vi "Motor Sets (SubVI).vi"() -> ()   [LabVIEW 2020]
uses:
  <vilib>/Rock Robotics/WPI/ThirdParty/Phoenix-LabVIEW/Motor Controller/Controls/CTRE_Phoenix_MotorControl_ControlMode.ctl
  <vilib>/Rock Robotics/WPI/ThirdParty/REV Robotics/REVLib/Typedef/Spark MAX Control Type.ctl
  <vilib>/Rock Robotics/WPI/ThirdParty/REV Robotics/REVLib/Typedef/Spark MAX Idle Mode.ctl
  Team Code/Robot Global Data.vi
  <vilib>/Rock Robotics/WPI/ThirdParty/Phoenix-LabVIEW/Motor Controller/Get/CTRE_Phoenix_MotorController_IntegratedSensorData_TalonFX.vi
  <vilib>/Rock Robotics/WPI/ThirdParty/Phoenix-LabVIEW/Motor Controller/Get/CTRE_Phoenix_MotorController_GetSelectedSensorData.vi
panel:
  in  "servoOverride":bool
  in  "servoPosition":dbl
  out "climerArmOutput":dbl
  in  "climberWinchOverride":bool
  in  "winchMode":T1=2 items=["PercentOutput"=0, "Position"=1, "Velocity"=2, "Current"=3, "Follower"=5, "MotionProfile"=6, "MotionMagic"=7, "MotionProfileArc"=10, "Disabled"=15]
  in  "winchOutput":dbl
  in  "kFWinch":dbl
  in  "kPWinch":dbl=0.06
  in  "kDWinch":dbl
  in  "climberWinchPIDOverride":bool
  out "climberWinch":dbl(graph)
  in  "climberArmOverride":bool
  out "climberArmPosition":dbl(graph)
  in  "climberArmControlMode":T2=enum."Position"
  in  "climberArmPosition":dbl
  in  "climberArmPIDConstants":T3={"P Gain"=0.01, "I Gain"=0.0, "D Gain"=0.0, "F Gain"=0.0, "I Zone"=0.0, "Min Output"=-0.5, "Max Output"=0.5}
  in  "climberArmPIDOveride":bool
  in  "intakeLift":bool
  out "intakeLiftPosition":dbl(graph)
  in  "intakeLiftControlMode":T2=enum."Position"
  in  "intakeLiftPosition":dbl
  in  "intakeLiftPIDConstants":T3={"P Gain"=0.0025, "I Gain"=0.0, "D Gain"=1.0, "F Gain"=0.0, "I Zone"=0.0, "Min Output"=-0.7, "Max Output"=0.7}
  in  "intakeLiftPIDOveride":bool
  in  "leftShooterOutput":dbl
  in  "intakeOverride":bool
  in  "intakeMode":T1 items=["PercentOutput"=0, "Position"=1, "Velocity"=2, "Current"=3, "Follower"=5, "MotionProfile"=6, "MotionMagic"=7, "MotionProfileArc"=10, "Disabled"=15]
  in  "intakeOutput":dbl
  in  "kFIntake":dbl=0.0491
  in  "kPIntake":dbl=0.06
  in  "kDIntake":dbl=5.0
  in  "intakePIDOverride":bool
  out "intake":i32(graph)
  out "turretAngle Position":dbl
  out "turretAngle":dbl(graph)
  in  "Turret PID Constants":T3={"P Gain"=0.0, "I Gain"=0.0, "D Gain"=0.0, "F Gain"=0.0, "I Zone"=0.0, "Min Output"=-1.0, "Max Output"=1.0}
  in  "hoodPIDOverride":bool
  in  "turretControlMotor":T2=enum."Position"
  in  "hoodPosition":dbl
  in  "PID Constants":T3={"P Gain"=0.009, "I Gain"=0.0, "D Gain"=0.0, "F Gain"=0.0, "I Zone"=0.0, "Min Output"=-0.6, "Max Output"=0.6}
  in  "Control Mode":T2=enum."Position"
  in  "kDShooter":dbl=2.0
  in  "kDKickup":dbl=5.0
  out "LoopTime (ms)":u32
  out "hoodAngle":dbl(graph)
  out "kickup":i32(graph)
  out "leftShooter":i32(graph)
  out "rightShooter":i32(graph)
  in  "turretAnglePIDOverride":bool
  in  "kickupPIDOverride":bool
  in  "kFKickup":dbl=0.0491
  in  "kPKickup":dbl=0.06
  in  "kPShooter":dbl=0.3
  in  "kFShooter":dbl=0.0506
  in  "shooterPIDOverride":bool
  in  "righrRearDriveOutput":dbl
  in  "leftRearDriveOutput":dbl
  in  "rightFrontDriveOutput":dbl
  out "rightRearDriveVelocity":i32(graph)
  out "leftRearDriveVelocity":i32(graph)
  out "rightFrontDriveVelocity":i32(graph)
  out "leftFrontDriveVelocity":i32(graph)
  in  "KdDrive":dbl
  in  "KpDrive":dbl
  in  "drivePIDOverride":bool
  in  "turretAngleOutput":dbl
  in  "turretAngleOverride":bool
  in  "hoodAngleOverride":bool
  in  "steeringMotorOverride":bool
  in  "rightRearSteeringOutput":dbl
  in  "leftRearSteeringOutput":dbl
  in  "rightFrontSteeringOutput":dbl
  in  "leftFrontSteeringOutput":dbl
  in  "indexerOutput":dbl
  in  "indexOverride":bool
  in  "driveMode":T1=2 items=["PercentOutput"=0, "Position"=1, "Velocity"=2, "Current"=3, "Follower"=5, "MotionProfile"=6, "MotionMagic"=7, "MotionProfileArc"=10, "Disabled"=15]
  in  "rightShooterOutput":dbl
  in  "shooterMode":T1=2 items=["PercentOutput"=0, "Position"=1, "Velocity"=2, "Current"=3, "Follower"=5, "MotionProfile"=6, "MotionMagic"=7, "MotionProfileArc"=10, "Disabled"=15]
  in  "shooterOverride":bool
  in  "kickupOutput":dbl
  in  "kickupMode":T1=2 items=["PercentOutput"=0, "Position"=1, "Velocity"=2, "Current"=3, "Follower"=5, "MotionProfile"=6, "MotionMagic"=7, "MotionProfileArc"=10, "Disabled"=15]
  in  "kickupOverride":bool
  in  "leftFrontDriveOutput":dbl
  in  "driveOverride":bool
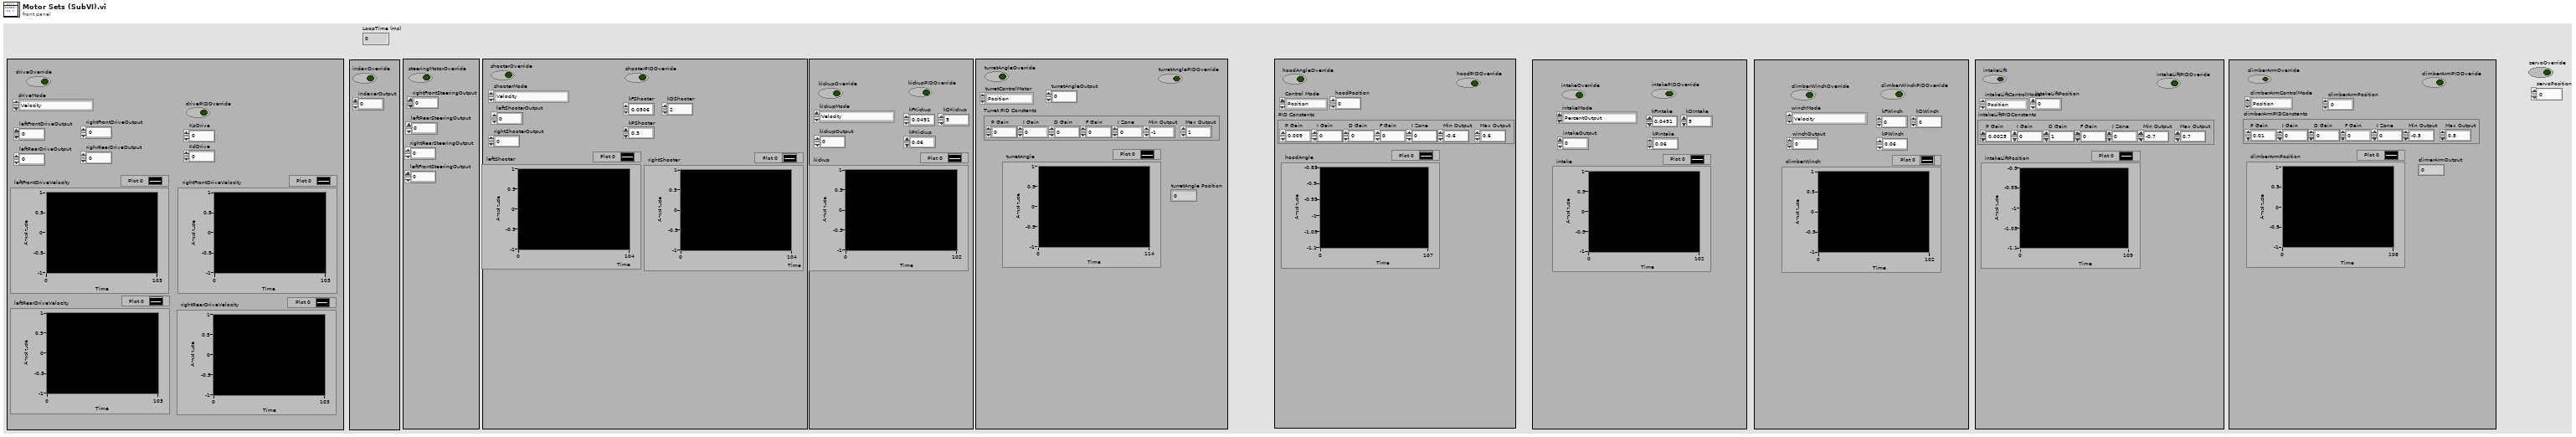
[diagram p1: front panel]
types:
  T1 = typedef "CTRE_Phoenix_MotorControl_ControlMode.ctl" = u16
  T2 = typedef "Spark MAX Control Type.ctl" = enum16{"Percent VBus", "Voltage", "Velocity", "Position", "Smart Motion", "Current", "Smart Velocity"}
  T3 = cluster{"P Gain":dbl, "I Gain":dbl, "D Gain":dbl, "F Gain":dbl, "I Zone":dbl, "Min Output":dbl, "Max Output":dbl}
  T4 = typedef "WPI_MotorControlDeviceRef.ctl" = cluster{"DeviceStatus":errorcluster, "Type":T5, "PWM":cluster{"PWM Channel":T6, "DeadBand":T7}, "CAN":cluster{"Device Number":u8, "SetOutput VI Ref":variant, "GetOutput VI Ref":variant, "Enable VI Ref":variant, "Disable VI Ref":variant, "Data":variant}, "Invert":bool, "DIO PWM":cluster{"PWM \"Enable\" Channel":T6, "DIOChannel":T8, "PWM Rate":dbl}}
  T5 = typedef "WPI_MotorControlType.ctl" = enum16{"PWM", "CAN", "DIO PWM"}
  T6 = typedef "FPGA_DIOPWMChannel.ctl" = enum8{"PWM 0", "PWM 1", "PWM 2", "PWM 3", "PWM 4", "PWM 5", "PWM 6", "PWM 7", "PWM 8", "PWM 9", "PWM MXP 0", "PWM MXP 1", "PWM MXP 2", "PWM MXP 3", "PWM MXP 4", "PWM MXP 5", "PWM MXP 6", "PWM MXP 7", "PWM MXP 8", "PWM MXP 9", "Invalid"}
  T7 = typedef "WPI_PWMDeadband.ctl" = cluster{"Name":string, "maxPositivePwm":i32, "minPositivePwm":i32, "centerPwm":i32, "maxNegativePwm":i32, "minNegativePwm":i32, "angularRange":u16}
  T8 = typedef "FPGA_DIOChannel.ctl" = enum8{"DIO 0", "DIO 1", "DIO 2", "DIO 3", "DIO 4", "DIO 5", "DIO 6", "DIO 7", "DIO 8", "DIO 9", "DIO MXP 0", "DIO MXP 1", "DIO MXP 2", "DIO MXP 3", "DIO MXP 4", "DIO MXP 5", "DIO MXP 6", "DIO MXP 7", "DIO MXP 8", "DIO MXP 9", "DIO MXP 10", "DIO MXP 11", "DIO MXP 12", "DIO MXP 13", "DIO MXP 14", "DIO MXP 15", "SPI Port CS1", "SPI Port CS2", "SPI Port CS3", "SPI Port MISO", "SPI Port MOSI", "Invalid"}
  T9 = typedef "WPI_ServoDeviceRef.ctl" = cluster{"DeviceStatus":errorcluster, "PWM Channel":T6, "DeadBand":T7}
  T10 = typedef "Spark MAX Idle Mode.ctl" = enum16{"Coast", "Brake"}
  T11 = cluster{"leftFrontDesiredVelocity":dbl, "leftRearDesiredVelocity":dbl, "rightFrontDesiredVelocity":dbl, "rightRearDesiredVelocity":dbl}
  T12 = cluster{"leftFrontSteeringPower":dbl, "leftRearSteeringPower":dbl, "rightFrontSteeringPower":dbl, "rightRearSteeringPower":dbl}
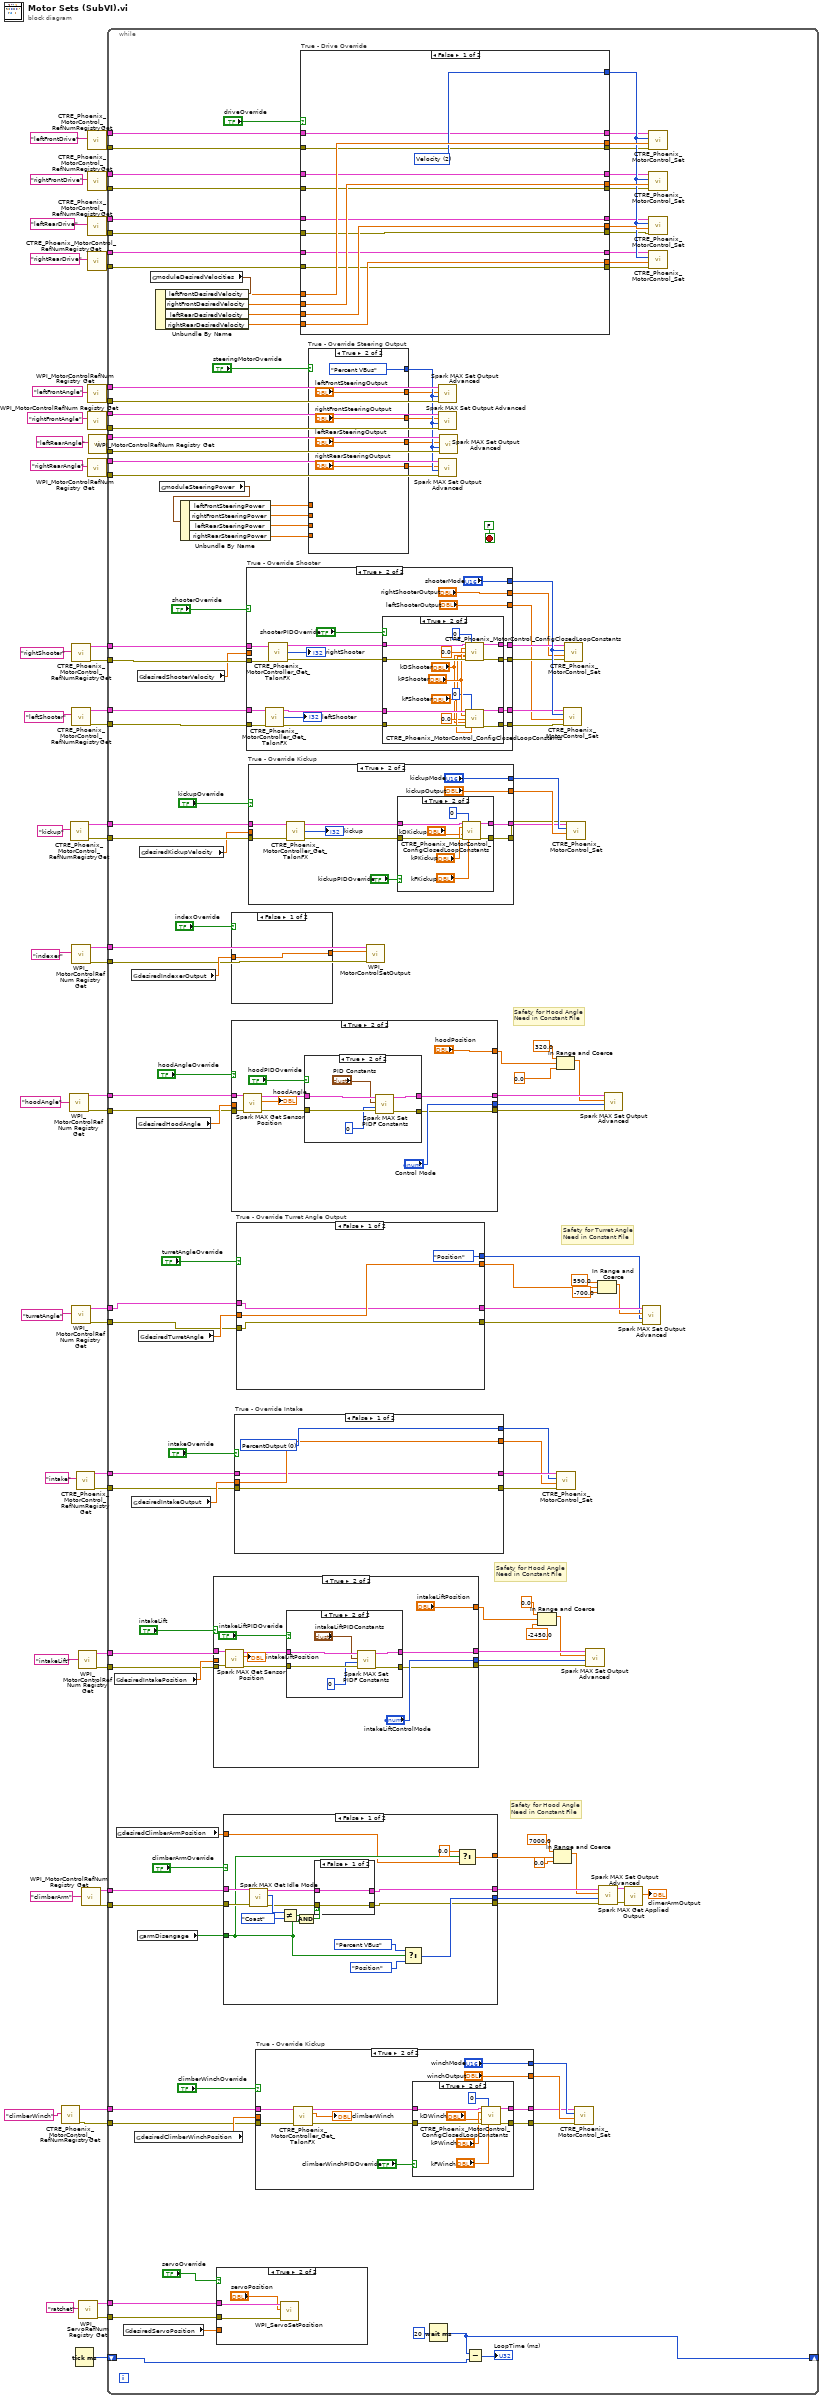
[diagram p0: block diagram]
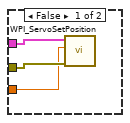
[diagram p2: hidden frame]
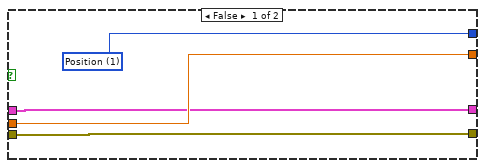
[diagram p3: hidden frame]
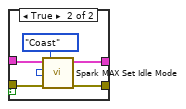
[diagram p5: hidden frame]
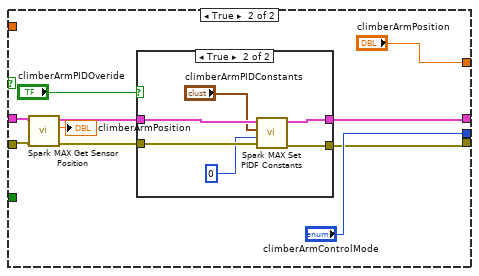
[diagram p6: hidden frame]
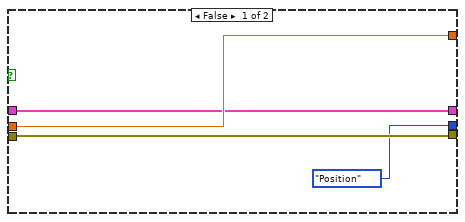
[diagram p8: hidden frame]
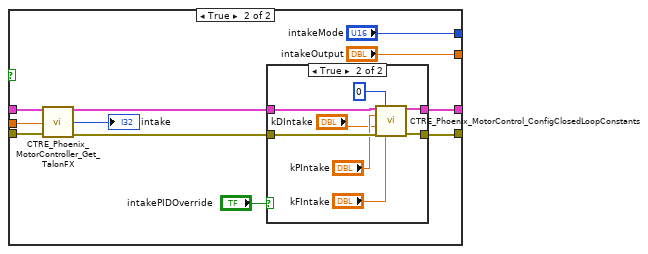
[diagram p10: hidden frame]
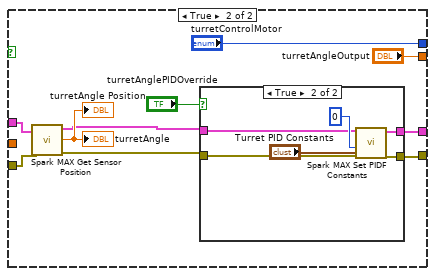
[diagram p12: hidden frame]
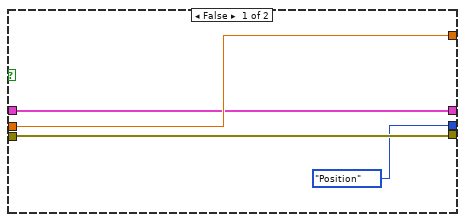
[diagram p14: hidden frame]
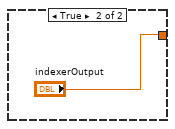
[diagram p16: hidden frame]
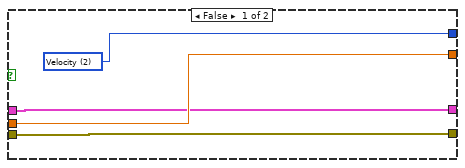
[diagram p17: hidden frame]
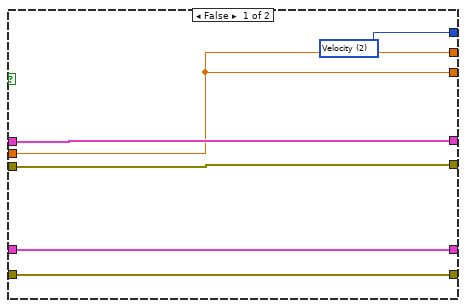
[diagram p19: hidden frame]
diagram:
  n1 = call <vilib>:"CTRE_Phoenix_MotorControl_RefNumRegistryGet.vi"("refnum name"="climberWinch") -> ("error out"=w4:errorcluster, "PhoenixMotorControlDevRef"=w5:T4)  [unwired: 9 in]
  n2 = call <vilib>:"WPI_MotorControlRefNum Registry Get.vi"("refnum name"="hoodAngle") -> ("error out"=w22:errorcluster, "MotorControlDevRef"=w23:T4)  [unwired: 9 in]
  n3 = call <vilib>:"CTRE_Phoenix_MotorControl_RefNumRegistryGet.vi"("refnum name"="kickup") -> ("error out"=w28:errorcluster, "PhoenixMotorControlDevRef"=w27:T4)  [unwired: 9 in]
  n4 = call <vilib>:"CTRE_Phoenix_MotorControl_RefNumRegistryGet.vi"("refnum name"="rightShooter") -> ("error out"=w30:errorcluster, "PhoenixMotorControlDevRef"=w29:T4)  [unwired: 9 in]
  n5 = call <vilib>:"CTRE_Phoenix_MotorControl_RefNumRegistryGet.vi"("refnum name"="leftShooter") -> ("error out"=w31:errorcluster, "PhoenixMotorControlDevRef"=w32:T4)  [unwired: 9 in]
  n6 = call <vilib>:"WPI_MotorControlRefNum Registry Get.vi"("refnum name"="indexer") -> ("error out"=w16:errorcluster, "MotorControlDevRef"=w17:T4)  [unwired: 9 in]
  n7 = call <vilib>:"WPI_MotorControlRefNum Registry Get.vi"("refnum name"="turretAngle") -> ("error out"=w19:errorcluster, "MotorControlDevRef"=w20:T4)  [unwired: 9 in]
  n8 = Tick Count (ms)() -> (millisecond timer value=w25:u32)
  n9 = call <vilib>:"CTRE_Phoenix_MotorControl_RefNumRegistryGet.vi"("refnum name"="intake") -> ("error out"=w13:errorcluster, "PhoenixMotorControlDevRef"=w14:T4)  [unwired: 9 in]
  n10 = call <vilib>:"WPI_MotorControlRefNum Registry Get.vi"("refnum name"="intakeLift") -> ("error out"=w10:errorcluster, "MotorControlDevRef"=w11:T4)  [unwired: 9 in]
  n11 = call <vilib>:"WPI_ServoRefNum Registry Get.vi"("refnum name"="ratchet") -> ("error out"=w1:errorcluster, "ServoDeviceRef"=w2:T9)  [unwired: 9 in]
  n12 = call <vilib>:"WPI_MotorControlRefNum Registry Get.vi"("refnum name"="climberArm") -> ("error out"=w7:errorcluster, "MotorControlDevRef"=w8:T4)  [unwired: 9 in]
  n13 = call <vilib>:"CTRE_Phoenix_MotorControl_RefNumRegistryGet.vi"("refnum name"="leftFrontDrive") -> ("error out"=w41:errorcluster, "PhoenixMotorControlDevRef"=w40:T4)  [unwired: 9 in]
  n14 = call <vilib>:"CTRE_Phoenix_MotorControl_RefNumRegistryGet.vi"("refnum name"="rightFrontDrive") -> ("error out"=w43:errorcluster, "PhoenixMotorControlDevRef"=w42:T4)  [unwired: 9 in]
  n15 = call <vilib>:"CTRE_Phoenix_MotorControl_RefNumRegistryGet.vi"("refnum name"="leftRearDrive") -> ("error out"=w45:errorcluster, "PhoenixMotorControlDevRef"=w44:T4)  [unwired: 9 in]
  n16 = call <vilib>:"CTRE_Phoenix_MotorControl_RefNumRegistryGet.vi"("refnum name"="rightRearDrive") -> ("error out"=w47:errorcluster, "PhoenixMotorControlDevRef"=w46:T4)  [unwired: 9 in]
  n17 = call <vilib>:"WPI_MotorControlRefNum Registry Get.vi"("refnum name"="leftFrontAngle") -> ("error out"=w49:errorcluster, "MotorControlDevRef"=w48:T4)  [unwired: 9 in]
  n18 = call <vilib>:"WPI_MotorControlRefNum Registry Get.vi"("refnum name"="rightFrontAngle") -> ("error out"=w50:errorcluster, "MotorControlDevRef"=w51:T4)  [unwired: 9 in]
  n19 = call <vilib>:"WPI_MotorControlRefNum Registry Get.vi"("refnum name"="rightRearAngle") -> ("error out"=w56:errorcluster, "MotorControlDevRef"=w57:T4)  [unwired: 9 in]
  n20 = call <vilib>:"WPI_MotorControlRefNum Registry Get.vi"("refnum name"="leftRearAngle") -> ("error out"=w55:errorcluster, "MotorControlDevRef"=w54:T4)  [unwired: 9 in]
  n21 = while {
    tunnel: w40 -> [w171]
    tunnel: w41 -> [w169]
    tunnel: w42 -> [w167]
    tunnel: w43 -> [w165]
    tunnel: w44 -> [w163]
    tunnel: w45 -> [w161]
    tunnel: w46 -> [w159]
    tunnel: w47 -> [w157]
    tunnel: w48 -> [w202]
    tunnel: w49 -> [w201]
    tunnel: w51 -> [w199]
    tunnel: w50 -> [w200]
    tunnel: w54 -> [w198]
    tunnel: w55 -> [w197]
    tunnel: w57 -> [w195]
    tunnel: w56 -> [w196]
    tunnel: w32 -> [w154]
    tunnel: w31 -> [w153]
    tunnel: w30 -> [w155]
    tunnel: w29 -> [w156]
    tunnel: w27 -> [w152]
    tunnel: w28 -> [w151]
    tunnel: w17 -> [w119]
    tunnel: w16 -> [w120]
    tunnel: w20 -> [w59]
    tunnel: w19 -> [w60]
    shift-right: [w147] -> _
    shift-left: w25 -> [w148]
    tunnel: w23 -> [w122]
    tunnel: w22 -> [w121]
    tunnel: w14 -> [w102]
    tunnel: w13 -> [w101]
    tunnel: w11 -> [w89]
    tunnel: w10 -> [w88]
    tunnel: w8 -> [w76]
    tunnel: w7 -> [w75]
    tunnel: w5 -> [w68]
    tunnel: w4 -> [w67]
    tunnel: w2 -> [w65]
    tunnel: w1 -> [w64]
    stop <- FALSE stop-if-true
    # "Safety for Hood Angle\nNeed in Constant File"
    # "Safety for Hood Angle\nNeed in Constant File"
    # "Safety for Turret Angle\nNeed in Constant File"
    # "Safety for Hood Angle\nNeed in Constant File"
    n22 = global read "Robot Global Data.vi" "desiredIntakePosition"() -> (w98:dbl)
    n23 = global read "Robot Global Data.vi" "desiredClimberArmPosition"() -> (w87:dbl)
    n24 = global read "Robot Global Data.vi" "desiredServoPosition"() -> (w62:dbl)
    n25 = global read "Robot Global Data.vi" "desiredIndexerOutput"() -> (w138:dbl)
    n26 = global read "Robot Global Data.vi" "desiredIntakeOutput"() -> (w104:dbl)
    n27 = global read "Robot Global Data.vi" "desiredClimberWinchPosition"() -> (w73:dbl)
    n28 = global read "Robot Global Data.vi" "desiredHoodAngle"() -> (w137:dbl)
    n29 = global read "Robot Global Data.vi" "desiredShooterVelocity"() -> (w145:dbl)
    n30 = global read "Robot Global Data.vi" "armDisengage"() -> (w61:bool)
    n31 = global read "Robot Global Data.vi" "desiredTurretAngle"() -> (w134:dbl)
    n32 = global read "Robot Global Data.vi" "desiredKickupVelocity"() -> (w143:dbl)
    n33 = global read "Robot Global Data.vi" "moduleDesiredVelocities"() -> (w192:T11)
    n34 = Unbundle By Name(w192) -> ("leftFrontDesiredVelocity"=w191:dbl, "rightFrontDesiredVelocity"=w190:dbl, "leftRearDesiredVelocity"=w189:dbl, "rightRearDesiredVelocity"=w188:dbl)
    n35 = global read "Robot Global Data.vi" "moduleSteeringPower"() -> (w193:T12)
    n36 = Unbundle By Name(w193) -> ("leftFrontSteeringPower"=w181:dbl, "rightFrontSteeringPower"=w180:dbl, "leftRearSteeringPower"=w179:dbl, "rightRearSteeringPower"=w178:dbl)
    n37 = case shown="True" "intakeLift" {
      tunnel: w98 -> [w279 _]
      tunnel: [w279 "intakeLiftPosition"] -> w96
      tunnel: w89 -> [w278 w280]
      tunnel: w88 -> [w277 w281]
      tunnel: [w277 w286] -> w92
      tunnel: [w278 w287] -> w93
      tunnel: [Spark_MAX_Control_Type."Position" ("Control Mode") "intakeLiftControlMode"] -> w90
      frame False {
      }
      frame True {
        n38 = call <vilib>:"Spark MAX Get Sensor Position.vi"("error in (no error)"=w281, "MotorControlDevRef in"=w280) -> ("error out"=w284:errorcluster, "Sensor Position"=→"intakeLiftPosition":dbl, "MotorControlDevRef out"=w285:T4)  [unwired: 6 in, 1 out]
        n39 = case shown="True" "intakeLiftPIDOveride" {
          tunnel: [w290 w297] -> w287
          tunnel: [w291 w296] -> w286
          tunnel: w285 -> [w290 w295]
          tunnel: w284 -> [w291 w294]
          frame False {
          }
          frame True {
            n40 = call <vilib>:"Spark MAX Set PIDF Constants.vi"("error in"=w294, "PIDF Slot"=0, "PID Constants"="intakeLiftPIDConstants", "MotorControlDeviceRef"=w295) -> ("error out"=w296:errorcluster, "MotorControlDeviceRef"=w297:T4)  [unwired: 6 in]
          }
        }
      }
    }
    n41 = case shown="True" "servoOverride" {
      tunnel: w65 -> [w206 w209]
      tunnel: w64 -> [w205 w208]
      tunnel: w62 -> [w204 _]
      frame False {
        n42 = call <vilib>:"WPI_ServoSetPosition.vi"("error in (no error)"=w205, "Position"=w204, "ServoDeviceRef"=w206) -> ()  [unwired: 7 in, 2 out]
      }
      frame True {
        n43 = call <vilib>:"WPI_ServoSetPosition.vi"("error in (no error)"=w208, "Position"="servoPosition", "ServoDeviceRef"=w209) -> ()  [unwired: 7 in, 2 out]
      }
    }
    n44 = case shown="False" "climberArmOverride" {
      tunnel: w87 -> [w235 _]
      tunnel: [w237 "climberArmPosition"] -> w85
      tunnel: w76 -> [w250 w258]
      tunnel: w75 -> [w249 w259]
      tunnel: [w238 w264] -> w79
      tunnel: [w239 w265] -> w80
      tunnel: [w242 "climberArmControlMode"] -> w77
      tunnel: w61 -> [w236 _]
      frame False {
        n45 = call <vilib>:"Spark MAX Get Idle Mode.vi"("error in (no error)"=w249, "MotorControlDeviceRef in"=w250) -> ("error out"=w243:errorcluster, "Idle Mode"=w248:T10, "MotorControlDeviceRef out"=w244:T4)  [unwired: 7 in]
        n46 = Not Equal?(x=w248, y=Spark_MAX_Idle_Mode."Coast") -> (x != y?=w246:bool)
        n47 = And(x=w246, y=w236) -> (x .and. y?=w245:bool)
        n48 = case shown="False" w245 {
          tunnel: w244 -> [w252 w256]
          tunnel: w243 -> [w251 w257]
          tunnel: [w252 w254] -> w239
          tunnel: [w251 w253] -> w238
          frame False {
          }
          frame True {
            n49 = call <vilib>:"Spark MAX Set Idle Mode.vi"("error in (no error)"=w257, "Idle Mode"=Spark_MAX_Idle_Mode."Coast", "MotorControlDeviceRef in"=w256) -> ("error out"=w253:errorcluster, "MotorControlDeviceRef out"=w254:T4)  [unwired: 7 in]
          }
        }
        n50 = Select(t=Spark_MAX_Control_Type."Percent VBus" ("Control Mode"), s=w236, f=Spark_MAX_Control_Type."Position" ("Control Mode")) -> (s? t:f=w242:T2)
        n51 = Select(t=0.0, s=w236, f=w235) -> (s? t:f=w237:dbl)
      }
      frame True {
        n52 = call <vilib>:"Spark MAX Get Sensor Position.vi"("error in (no error)"=w259, "MotorControlDevRef in"=w258) -> ("error out"=w262:errorcluster, "Sensor Position"=→"climberArmPosition":dbl, "MotorControlDevRef out"=w263:T4)  [unwired: 6 in, 1 out]
        n53 = case shown="True" "climberArmPIDOveride" {
          tunnel: [w268 w275] -> w265
          tunnel: [w269 w274] -> w264
          tunnel: w263 -> [w268 w273]
          tunnel: w262 -> [w269 w272]
          frame False {
          }
          frame True {
            n54 = call <vilib>:"Spark MAX Set PIDF Constants.vi"("error in"=w272, "PIDF Slot"=0, "PID Constants"="climberArmPIDConstants", "MotorControlDeviceRef"=w273) -> ("error out"=w274:errorcluster, "MotorControlDeviceRef"=w275:T4)  [unwired: 6 in]
          }
        }
      }
    }
    n55 = case shown="False" "indexOverride" {
      tunnel: w138 -> [w367 _]
      tunnel: [w367 "indexerOutput"] -> w118
      frame False {
      }
      frame True {
      }
    }
    n56 = case shown="True" "hoodAngleOverride" {
      tunnel: w137 -> [w348 _]
      tunnel: [w348 "hoodPosition"] -> w127
      tunnel: w122 -> [w347 w358]
      tunnel: w121 -> [w346 w357]
      tunnel: [w346 w353] -> w116
      tunnel: [w347 w354] -> w117
      tunnel: [Spark_MAX_Control_Type."Position" ("Control Mode") "Control Mode"] -> w114
      frame False {
      }
      frame True {
        n57 = call <vilib>:"Spark MAX Get Sensor Position.vi"("error in (no error)"=w357, "MotorControlDevRef in"=w358) -> ("error out"=w351:errorcluster, "Sensor Position"=→"hoodAngle":dbl, "MotorControlDevRef out"=w352:T4)  [unwired: 6 in, 1 out]
        n58 = case shown="True" "hoodPIDOverride" {
          tunnel: [w359 w366] -> w354
          tunnel: [w360 w365] -> w353
          tunnel: w352 -> [w359 w364]
          tunnel: w351 -> [w360 w363]
          frame False {
          }
          frame True {
            n59 = call <vilib>:"Spark MAX Set PIDF Constants.vi"("error in"=w363, "PIDF Slot"=0, "PID Constants"="PID Constants", "MotorControlDeviceRef"=w364) -> ("error out"=w365:errorcluster, "MotorControlDeviceRef"=w366:T4)  [unwired: 6 in]
          }
        }
      }
    }
    n60 = case "True - Override Intake" shown="False" "intakeOverride" {
      tunnel: [w301 "intakeMode"] -> w103
      tunnel: w104 -> [w300 w310]
      tunnel: [w300 "intakeOutput"] -> w105
      tunnel: [w299 w307] -> w107
      tunnel: [w298 w306] -> w108
      tunnel: w102 -> [w299 w303]
      tunnel: w101 -> [w298 w302]
      frame False {
        w301 = T1 0 items=["PercentOutput"=0, "Position"=1, "Velocity"=2, "Current"=3, "Follower"=5, "MotionProfile"=6, "MotionMagic"=7, "MotionProfileArc"=10, "Disabled"=15] ("Control Mode")
      }
      frame True {
        n61 = call-poly <vilib>:"CTRE_Phoenix_MotorController_Get_TalonFX.vi"("PhoenixMotorControlDevRef"=w303, "pidLoopIdx"=w310, "error in"=w302) -> ("PhoenixMotorControlDevRef"=w309:T4, "Velocity (Raw Sensor Units per 100 ms)"=→"intake":i32, "error out"=w308:errorcluster)  [unwired: 9 in, 1 out]
        n62 = case shown="True" "intakePIDOverride" {
          tunnel: [w314 w320] -> w307
          tunnel: w309 -> [w314 w322]
          tunnel: [w313 w319] -> w306
          tunnel: w308 -> [w313 w321]
          frame False {
          }
          frame True {
            n63 = call <vilib>:"CTRE_Phoenix_MotorControl_ConfigClosedLoopConstants.vi"("PhoenixMotorControlDevRef"=w322, "slotIdx"=0, "P"="kPIntake", "D"="kDIntake", "error in (no error)"=w321, "F"="kFIntake") -> ("PhoenixMotorControlDevRef"=w320:T4, "error out"=w319:errorcluster)  [unwired: 8 in]
          }
        }
      }
    }
    n64 = case "True - Override Turret Angle Output" shown="False" "turretAngleOverride" {
      tunnel: w134 -> [w326 _]
      tunnel: [w326 "turretAngleOutput"] -> w124
      tunnel: [w324 w335] -> w113
      tunnel: [w323 w334] -> w112
      tunnel: [Spark_MAX_Control_Type."Position" ("turretControlMotor") "turretControlMotor"] -> w110
      tunnel: w60 -> [w323 w330]
      tunnel: w59 -> [w324 w329]
      frame False {
      }
      frame True {
        n65 = call <vilib>:"Spark MAX Get Sensor Position.vi"("error in (no error)"=w330, "MotorControlDevRef in"=w329) -> ("error out"=w328:errorcluster, "Sensor Position"=→"turretAngle" →"turretAngle Position":dbl, "MotorControlDevRef out"=w327:T4)  [unwired: 6 in, 1 out]
        n66 = case shown="True" "turretAnglePIDOverride" {
          tunnel: w327 -> [w338 w343]
          tunnel: [w338 w342] -> w335
          tunnel: w328 -> [w337 w340]
          tunnel: [w337 w341] -> w334
          frame False {
          }
          frame True {
            n67 = call <vilib>:"Spark MAX Set PIDF Constants.vi"("error in"=w340, "PIDF Slot"=0 ("slotIdx"), "PID Constants"="Turret PID Constants", "MotorControlDeviceRef"=w343) -> ("error out"=w341:errorcluster, "MotorControlDeviceRef"=w342:T4)  [unwired: 6 in]
          }
        }
      }
    }
    n68 = case "True - Override Shooter" shown="True" "shooterOverride" {
      tunnel: [w398 "shooterMode"] -> w146
      tunnel: w145 -> [w393 _]
      tunnel: [w393 "rightShooterOutput"] -> w109
      tunnel: [w397 w413] -> w133
      tunnel: w156 -> [w397 w414]
      tunnel: [w396 w410] -> w132
      tunnel: w155 -> [w396 w411]
      tunnel: [w395 w406] -> w131
      tunnel: w154 -> [w395 w408]
      tunnel: [w394 w404] -> w130
      tunnel: w153 -> [w394 w407]
      tunnel: [w393 "leftShooterOutput"] -> w99
      frame False {
        w398 = T1 2 items=["PercentOutput"=0, "Position"=1, "Velocity"=2, "Current"=3, "Follower"=5, "MotionProfile"=6, "MotionMagic"=7, "MotionProfileArc"=10, "Disabled"=15] ("Control Mode")
      }
      frame True {
        n69 = call-poly <vilib>:"CTRE_Phoenix_MotorController_Get_TalonFX.vi"("PhoenixMotorControlDevRef"=w408, "error in"=w407) -> ("PhoenixMotorControlDevRef"=w405:T4, "Velocity (Raw Sensor Units per 100 ms)"=→"leftShooter":i32, "error out"=w403:errorcluster)  [unwired: 10 in, 1 out]
        n70 = call-poly <vilib>:"CTRE_Phoenix_MotorController_Get_TalonFX.vi"("PhoenixMotorControlDevRef"=w414, "error in"=w411) -> ("PhoenixMotorControlDevRef"=w412:T4, "Velocity (Raw Sensor Units per 100 ms)"=→"rightShooter":i32, "error out"=w409:errorcluster)  [unwired: 10 in, 1 out]
        n71 = case shown="True" "shooterPIDOverride" {
          tunnel: [w420 w433] -> w413
          tunnel: w412 -> [w420 w435]
          tunnel: [w419 w432] -> w410
          tunnel: w409 -> [w419 w434]
          tunnel: [w418 w429] -> w406
          tunnel: w405 -> [w418 w431]
          tunnel: [w417 w428] -> w404
          tunnel: w403 -> [w417 w430]
          frame False {
          }
          frame True {
            n72 = call <vilib>:"CTRE_Phoenix_MotorControl_ConfigClosedLoopConstants.vi"("PhoenixMotorControlDevRef"=w435, "slotIdx"=0, "P"="kPShooter", "I"=0.0, "D"="kDShooter", "error in (no error)"=w434, "F"="kFShooter") -> ("PhoenixMotorControlDevRef"=w433:T4, "error out"=w432:errorcluster)  [unwired: 7 in]
            n73 = call <vilib>:"CTRE_Phoenix_MotorControl_ConfigClosedLoopConstants.vi"("PhoenixMotorControlDevRef"=w431, "slotIdx"=0, "P"="kPShooter", "I"=0.0, "D"="kDShooter", "error in (no error)"=w430, "F"="kFShooter") -> ("PhoenixMotorControlDevRef"=w429:T4, "error out"=w428:errorcluster)  [unwired: 7 in]
          }
        }
      }
    }
    n74 = case "True - Override Kickup" shown="True" "kickupOverride" {
      tunnel: [w372 "kickupMode"] -> w144
      tunnel: w143 -> [w371 _]
      tunnel: [w371 "kickupOutput"] -> w142
      tunnel: [w370 w376] -> w129
      tunnel: w152 -> [w370 w378]
      tunnel: [w369 w375] -> w128
      tunnel: w151 -> [w369 w377]
      frame False {
        w372 = T1 2 items=["PercentOutput"=0, "Position"=1, "Velocity"=2, "Current"=3, "Follower"=5, "MotionProfile"=6, "MotionMagic"=7, "MotionProfileArc"=10, "Disabled"=15] ("Control Mode")
      }
      frame True {
        n75 = call-poly <vilib>:"CTRE_Phoenix_MotorController_Get_TalonFX.vi"("PhoenixMotorControlDevRef"=w378, "error in"=w377) -> ("PhoenixMotorControlDevRef"=w380:T4, "Velocity (Raw Sensor Units per 100 ms)"=→"kickup":i32, "error out"=w379:errorcluster)  [unwired: 10 in, 1 out]
        n76 = case shown="True" "kickupPIDOverride" {
          tunnel: [w384 w390] -> w376
          tunnel: w380 -> [w384 w392]
          tunnel: [w383 w389] -> w375
          tunnel: w379 -> [w383 w391]
          frame False {
          }
          frame True {
            n77 = call <vilib>:"CTRE_Phoenix_MotorControl_ConfigClosedLoopConstants.vi"("PhoenixMotorControlDevRef"=w392, "slotIdx"=0, "P"="kPKickup", "D"="kDKickup", "error in (no error)"=w391, "F"="kFKickup") -> ("PhoenixMotorControlDevRef"=w390:T4, "error out"=w389:errorcluster)  [unwired: 8 in]
          }
        }
      }
    }
    n78 = case "True - Override Kickup" shown="True" "climberWinchOverride" {
      tunnel: [w213 "winchMode"] -> w74
      tunnel: w73 -> [w212 _]
      tunnel: [w212 "winchOutput"] -> w72
      tunnel: [w211 w217] -> w70
      tunnel: w68 -> [w211 w219]
      tunnel: [w210 w216] -> w69
      tunnel: w67 -> [w210 w218]
      frame False {
        w213 = T1 1 items=["PercentOutput"=0, "Position"=1, "Velocity"=2, "Current"=3, "Follower"=5, "MotionProfile"=6, "MotionMagic"=7, "MotionProfileArc"=10, "Disabled"=15] ("Control Mode")
      }
      frame True {
        n79 = call-poly <vilib>:"CTRE_Phoenix_MotorController_Get_TalonFX.vi"("PhoenixMotorControlDevRef"=w219, "error in"=w218) -> ("PhoenixMotorControlDevRef"=w221:T4, "Position"=→"climberWinch":dbl, "error out"=w220:errorcluster)  [unwired: 9 in, 2 out]
        n80 = case shown="True" "climberWinchPIDOverride" {
          tunnel: [w225 w231] -> w217
          tunnel: w221 -> [w225 w233]
          tunnel: [w224 w230] -> w216
          tunnel: w220 -> [w224 w232]
          frame False {
          }
          frame True {
            n81 = call <vilib>:"CTRE_Phoenix_MotorControl_ConfigClosedLoopConstants.vi"("PhoenixMotorControlDevRef"=w233, "slotIdx"=0, "P"="kPWinch", "D"="kDWinch", "error in (no error)"=w232, "F"="kFWinch") -> ("PhoenixMotorControlDevRef"=w231:T4, "error out"=w230:errorcluster)  [unwired: 8 in]
          }
        }
      }
    }
    n82 = case "True - Drive Override" shown="False" "driveOverride" {
      tunnel: w191 -> [w458 _]
      tunnel: w190 -> [w457 _]
      tunnel: w189 -> [w456 _]
      tunnel: w188 -> [w455 _]
      tunnel: [w458 "leftFrontDriveOutput"] -> w187
      tunnel: [w457 "rightFrontDriveOutput"] -> w186
      tunnel: [w456 "leftRearDriveOutput"] -> w185
      tunnel: [w455 "righrRearDriveOutput"] -> w184
      tunnel: [w454 "driveMode"] -> w182
      tunnel: [w453 w480] -> w172
      tunnel: w171 -> [w453 w490]
      tunnel: [w452 w479] -> w170
      tunnel: w169 -> [w452 w491]
      tunnel: [w451 w478] -> w168
      tunnel: w167 -> [w451 w489]
      tunnel: [w450 w476] -> w166
      tunnel: w165 -> [w450 w488]
      tunnel: [w449 w474] -> w164
      tunnel: w163 -> [w449 w484]
      tunnel: [w448 w472] -> w162
      tunnel: w161 -> [w448 w487]
      tunnel: [w447 w470] -> w160
      tunnel: w159 -> [w447 w486]
      tunnel: [w446 w468] -> w158
      tunnel: w157 -> [w446 w485]
      frame False {
        w454 = T1 2 items=["PercentOutput"=0, "Position"=1, "Velocity"=2, "Current"=3, "Follower"=5, "MotionProfile"=6, "MotionMagic"=7, "MotionProfileArc"=10, "Disabled"=15] ("Control Mode")
      }
      frame True {
        n83 = call-poly <vilib>:"CTRE_Phoenix_MotorController_Get_TalonFX.vi"("PhoenixMotorControlDevRef"=w490, "error in"=w491) -> ("PhoenixMotorControlDevRef"=w482:T4, "Velocity (Raw Sensor Units per 100 ms)"=→"leftFrontDriveVelocity":i32, "error out"=w481:errorcluster)  [unwired: 10 in, 1 out]
        n84 = call-poly <vilib>:"CTRE_Phoenix_MotorController_Get_TalonFX.vi"("PhoenixMotorControlDevRef"=w489, "error in"=w488) -> ("PhoenixMotorControlDevRef"=w477:T4, "Velocity (Raw Sensor Units per 100 ms)"=→"rightFrontDriveVelocity":i32, "error out"=w475:errorcluster)  [unwired: 10 in, 1 out]
        n85 = call-poly <vilib>:"CTRE_Phoenix_MotorController_Get_TalonFX.vi"("PhoenixMotorControlDevRef"=w484, "error in"=w487) -> ("PhoenixMotorControlDevRef"=w473:T4, "Velocity (Raw Sensor Units per 100 ms)"=→"leftRearDriveVelocity":i32, "error out"=w471:errorcluster)  [unwired: 10 in, 1 out]
        n86 = call-poly <vilib>:"CTRE_Phoenix_MotorController_Get_TalonFX.vi"("PhoenixMotorControlDevRef"=w486, "error in"=w485) -> ("PhoenixMotorControlDevRef"=w469:T4, "Velocity (Raw Sensor Units per 100 ms)"=→"rightRearDriveVelocity":i32, "error out"=w467:errorcluster)  [unwired: 10 in, 1 out]
        n87 = case "True - PID Override" shown="True" "drivePIDOverride" {
          tunnel: w482 -> [w500 w519]
          tunnel: w481 -> [w499 w518]
          tunnel: [w500 w517] -> w480
          tunnel: [w499 w516] -> w479
          tunnel: [w498 w510] -> w478
          tunnel: w477 -> [w498 w512]
          tunnel: [w497 w515] -> w476
          tunnel: w475 -> [w497 w511]
          tunnel: [w496 w509] -> w474
          tunnel: w473 -> [w496 w508]
          tunnel: [w495 w514] -> w472
          tunnel: w471 -> [w495 w507]
          tunnel: [w494 w513] -> w470
          tunnel: w469 -> [w494 w506]
          tunnel: [w493 w504] -> w468
          tunnel: w467 -> [w493 w505]
          frame False {
          }
          frame True {
            w501 = 0 ("slotIdx")
            n88 = call <vilib>:"CTRE_Phoenix_MotorControl_ConfigClosedLoopConstants.vi"("PhoenixMotorControlDevRef"=w519, "slotIdx"=w501, "P"="KpDrive", "D"="KdDrive", "error in (no error)"=w518) -> ("PhoenixMotorControlDevRef"=w517:T4, "error out"=w516:errorcluster)  [unwired: 9 in]
            n89 = call <vilib>:"CTRE_Phoenix_MotorControl_ConfigClosedLoopConstants.vi"("PhoenixMotorControlDevRef"=w512, "slotIdx"=w501, "P"="KpDrive", "D"="KdDrive", "error in (no error)"=w511) -> ("PhoenixMotorControlDevRef"=w510:T4, "error out"=w515:errorcluster)  [unwired: 9 in]
            n90 = call <vilib>:"CTRE_Phoenix_MotorControl_ConfigClosedLoopConstants.vi"("PhoenixMotorControlDevRef"=w508, "slotIdx"=w501, "P"="KpDrive", "D"="KdDrive", "error in (no error)"=w507) -> ("PhoenixMotorControlDevRef"=w509:T4, "error out"=w514:errorcluster)  [unwired: 9 in]
            n91 = call <vilib>:"CTRE_Phoenix_MotorControl_ConfigClosedLoopConstants.vi"("PhoenixMotorControlDevRef"=w506, "slotIdx"=w501, "P"="KpDrive", "D"="KdDrive", "error in (no error)"=w505) -> ("PhoenixMotorControlDevRef"=w513:T4, "error out"=w504:errorcluster)  [unwired: 9 in]
          }
        }
      }
    }
    n92 = case "True - Override Steering Output" shown="True" "steeringMotorOverride" {
      tunnel: [Spark_MAX_Control_Type."Percent VBus" ("Control Mode") Spark_MAX_Control_Type."Percent VBus" ("Control Mode")] -> w194
      tunnel: w181 -> [w439 _]
      tunnel: w180 -> [w438 _]
      tunnel: w179 -> [w437 _]
      tunnel: w178 -> [w436 _]
      tunnel: [w439 "leftFrontSteeringOutput"] -> w177
      tunnel: [w438 "rightFrontSteeringOutput"] -> w176
      tunnel: [w437 "leftRearSteeringOutput"] -> w175
      tunnel: [w436 "rightRearSteeringOutput"] -> w174
      frame False {
      }
      frame True {
      }
    }
    n93 = call <vilib>:"WPI_MotorControlSetOutput.vi"("error in (no error)"=w120, "Output"=w118, "MotorControlDevRef"=w119) -> ()  [unwired: 6 in, 3 out]
    n94 = Wait (ms)(milliseconds to wait=u32 20) -> (millisecond timer value=w147:u32)
    n95 = call <vilib>:"Spark MAX Set Output Advanced.vi"("error in (no error)"=w201, "Control Mode"=w194, "Setpoint"=w177, "MotorControlDevRef"=w202) -> ()  [unwired: 6 in, 2 out]
    n96 = call <vilib>:"Spark MAX Set Output Advanced.vi"("error in (no error)"=w200, "Control Mode"=w194, "Setpoint"=w176, "MotorControlDevRef"=w199) -> ()  [unwired: 6 in, 2 out]
    n97 = call <vilib>:"Spark MAX Set Output Advanced.vi"("error in (no error)"=w196, "Control Mode"=w194, "Setpoint"=w174, "MotorControlDevRef"=w195) -> ()  [unwired: 6 in, 2 out]
    n98 = call <vilib>:"Spark MAX Set Output Advanced.vi"("error in (no error)"=w197, "Control Mode"=w194, "Setpoint"=w175, "MotorControlDevRef"=w198) -> ()  [unwired: 6 in, 2 out]
    n99 = Subtract(x=w147, y=w148) -> (x-y=→"LoopTime (ms)":u32)
    n100 = In Range and Coerce(upper limit=0.0, x=w96, lower limit=-2450.0) -> (coerced(x)=w91:dbl)  [unwired: 1 out]
    n101 = In Range and Coerce(upper limit=7000.0, x=w85, lower limit=0.0) -> (coerced(x)=w78:dbl)  [unwired: 1 out]
    n102 = In Range and Coerce(upper limit=320.0, x=w127, lower limit=0.0) -> (coerced(x)=w115:dbl)  [unwired: 1 out]
    n103 = call <vilib>:"CTRE_Phoenix_MotorControl_Set.vi"("error in (no error)"=w108, "Output"=w105, "Control Mode"=w103, "PhoenixMotorControlDevRef"=w107) -> ()  [unwired: 6 in, 2 out]
    n104 = call <vilib>:"CTRE_Phoenix_MotorControl_Set.vi"("error in (no error)"=w130, "Output"=w99, "Control Mode"=w146, "PhoenixMotorControlDevRef"=w131) -> ()  [unwired: 6 in, 2 out]
    n105 = call <vilib>:"CTRE_Phoenix_MotorControl_Set.vi"("error in (no error)"=w132, "Output"=w109, "Control Mode"=w146, "PhoenixMotorControlDevRef"=w133) -> ()  [unwired: 6 in, 2 out]
    n106 = call <vilib>:"CTRE_Phoenix_MotorControl_Set.vi"("error in (no error)"=w128, "Output"=w142, "Control Mode"=w144, "PhoenixMotorControlDevRef"=w129) -> ()  [unwired: 6 in, 2 out]
    n107 = call <vilib>:"CTRE_Phoenix_MotorControl_Set.vi"("error in (no error)"=w69, "Output"=w72, "Control Mode"=w74, "PhoenixMotorControlDevRef"=w70) -> ()  [unwired: 6 in, 2 out]
    n108 = call <vilib>:"Spark MAX Set Output Advanced.vi"("error in (no error)"=w92, "Control Mode"=w90, "Setpoint"=w91, "MotorControlDevRef"=w93) -> ()  [unwired: 6 in, 2 out]
    n109 = In Range and Coerce(upper limit=590.0, x=w124, lower limit=-700.0) -> (coerced(x)=w111:dbl)  [unwired: 1 out]
    n110 = call <vilib>:"Spark MAX Set Output Advanced.vi"("error in (no error)"=w79, "Control Mode"=w77, "Setpoint"=w78, "MotorControlDevRef"=w80) -> ("error out"=w81:errorcluster, "MotorControlDevRef"=w82:T4)  [unwired: 6 in]
    n111 = call <vilib>:"Spark MAX Set Output Advanced.vi"("error in (no error)"=w116, "Control Mode"=w114, "Setpoint"=w115, "MotorControlDevRef"=w117) -> ()  [unwired: 6 in, 2 out]
    n112 = call <vilib>:"Spark MAX Get Applied Output.vi"("error in (no error)"=w81, "MotorControlDevRef in"=w82) -> ("Applied Output"=→"climerArmOutput":dbl)  [unwired: 6 in, 3 out]
    n113 = call <vilib>:"Spark MAX Set Output Advanced.vi"("error in (no error)"=w112, "Control Mode"=w110, "Setpoint"=w111, "MotorControlDevRef"=w113) -> ()  [unwired: 6 in, 2 out]
    n114 = call <vilib>:"CTRE_Phoenix_MotorControl_Set.vi"("error in (no error)"=w170, "Output"=w187, "Control Mode"=w182, "PhoenixMotorControlDevRef"=w172) -> ()  [unwired: 6 in, 2 out]
    n115 = call <vilib>:"CTRE_Phoenix_MotorControl_Set.vi"("error in (no error)"=w166, "Output"=w186, "Control Mode"=w182, "PhoenixMotorControlDevRef"=w168) -> ()  [unwired: 6 in, 2 out]
    n116 = call <vilib>:"CTRE_Phoenix_MotorControl_Set.vi"("error in (no error)"=w162, "Output"=w185, "Control Mode"=w182, "PhoenixMotorControlDevRef"=w164) -> ()  [unwired: 6 in, 2 out]
    n117 = call <vilib>:"CTRE_Phoenix_MotorControl_Set.vi"("error in (no error)"=w158, "Output"=w184, "Control Mode"=w182, "PhoenixMotorControlDevRef"=w160) -> ()  [unwired: 6 in, 2 out]
  }
